vi "VoltageTest_L.vi"(0 "datain":string[](array[string])=["备注", "负载通道", "负载地址", "延时时间", "output max", "output min", "量测类型", "待测物板号"], 5 "HW CH Number":i32=4, 7 "Setup":string) -> (4 "REPORT INDECATE":string[][](array[string])=[["微安测试", "", "", "", ""], ["微安量测", "4", "0.000", "0.1", "NG"], ["微安量测", "4", "0.000", "0.1", "NG"], ["微安量测", "4", "0.000", "0.1", "NG"], ["微安量测", "4", "0.000", "0.1", "NG"]], 6 "ROW HEAD":string[](array[string]), 8 "PF":string[](array[string]), 10 "testData":string[](array[string]), 14 "数组":bool[](array[boolean]), 15 "Array":string[](array[string]))   [LabVIEW 2018]
uses:
  Subvi/Global.vi
panel:
  out "测试板数":i32=4
  # "[VoltageTest]\nExt.Name =2222222222;\nAddress =1;\nDelay Time =1;\nMAX.Spec =*;\nMin.Spec =2;\nTest Type =;\nRelayH_8Bit =0,0,0,0;\nRelayL_8Bit =0,0,0,0;\nStart board number =1;#"
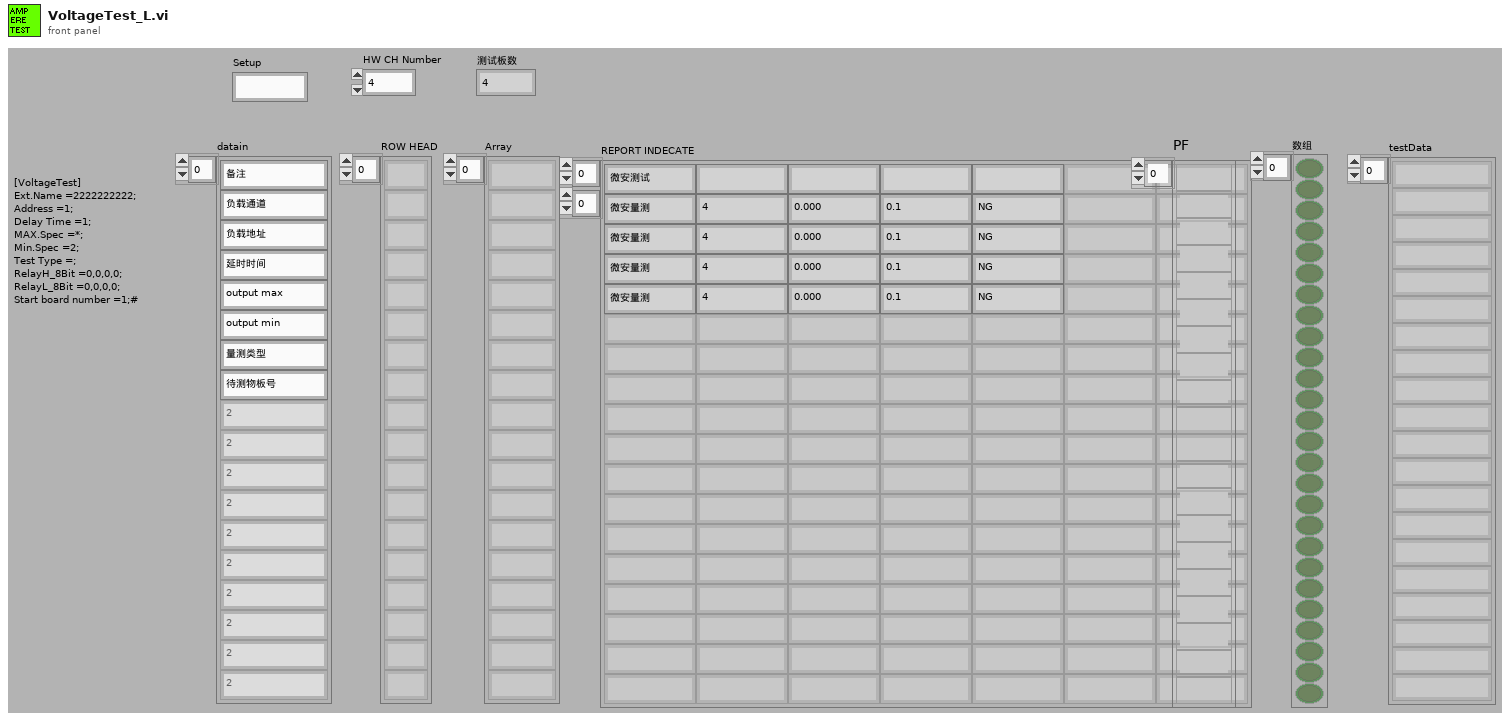
[diagram p1: front panel]
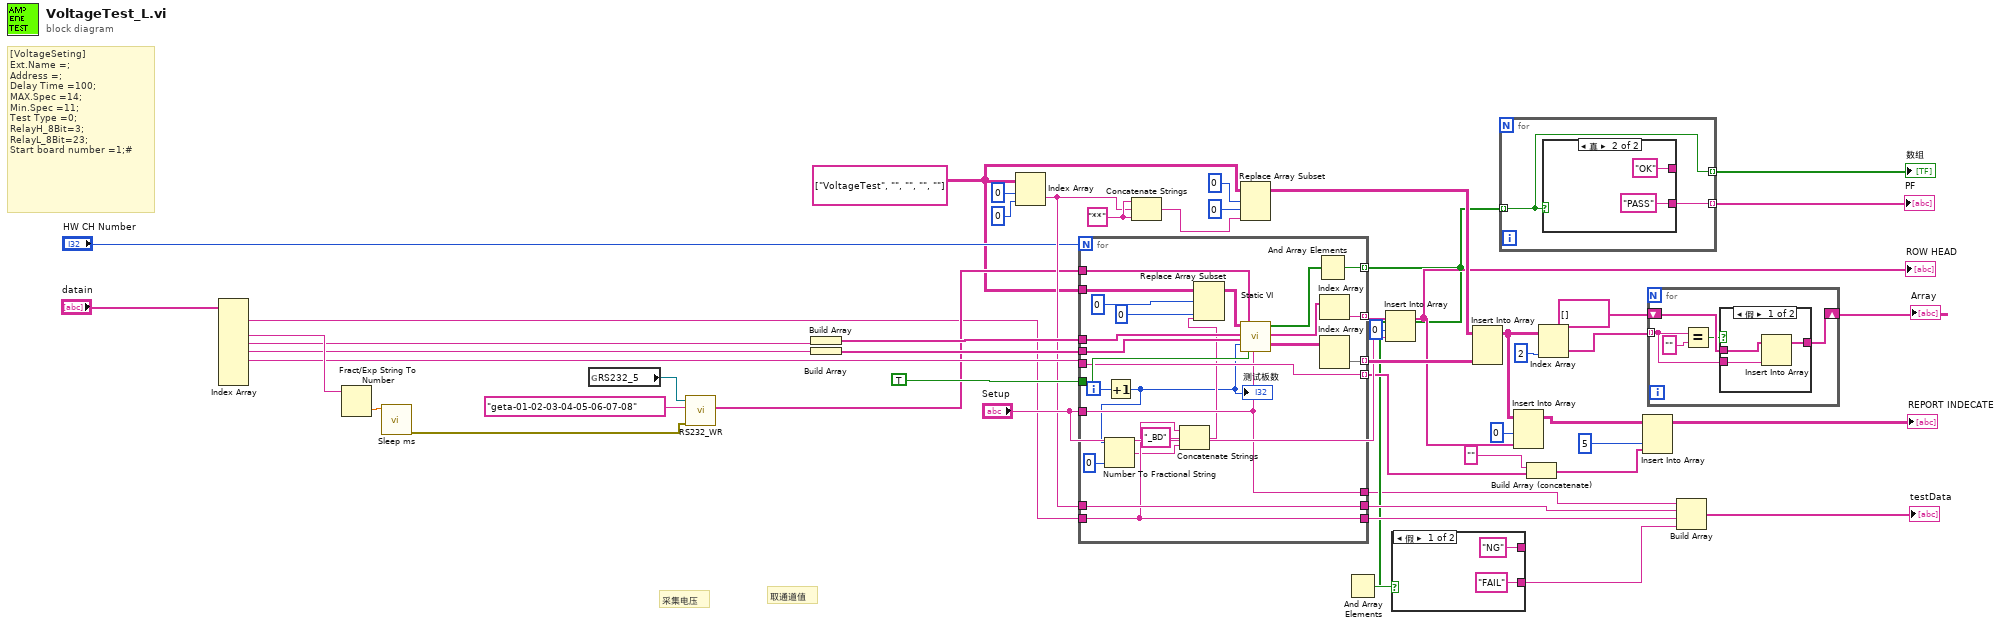
[diagram p0: block diagram]
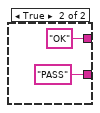
[diagram p2: hidden frame]
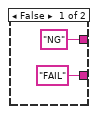
[diagram p3: hidden frame]
diagram:
  w5 = string[][] [["VoltageTest", "", "", "", ""]]
  w41 = "**" ("字符串")
  # "取通道值"
  # "采集电压"
  # "[VoltageSeting]\nExt.Name =;\nAddress =;\nDelay Time =100;\nMAX.Spec =14;\nMin.Spec =11;\nTest Type =0;\nRelayH_8Bit=3;\nRelayL_8Bit=23;\nStart board number =1;#"
  n1 = Index Array(array="datain") -> (element #1=w6:string, element #3=w44:string, element #4=w37:string, element #5=w36:string, element #6=w24:string)  [unwired: 9 in, 4 out]
  n2 = Fract/Exp String To Number(string=w44) -> (number=w2:dbl)  [unwired: 3 in, 1 out]
  n3 = call "Sleep ms.vi"("等待时间（毫秒）"=w2) -> ("error out"=w1:errorcluster)  [unwired: 10 in]
  n4 = global read "Global.vi" "RS232_5"() -> (w3:refnum<visa-resource-name>)
  n5 = call "RS232_WR.vi"("error in (no error)"=w1, "CMD"="geta-01-02-03-04-05-06-07-08", "VISA资源名称"=w3) -> ("Out data"=w7:string[])  [unwired: 6 in, 2 out]
  n6 = Build Array(w37) -> (w35:string[])
  n7 = Build Array(w36) -> (w34:string[])
  n8 = Index Array(array=w5, index (row)=0 ("索引 (行)"), index (col)=0 ("禁用的索引 (列)")) -> (element=w17:string)
  n9 = for {
    N: "HW CH Number" -> [_]
    tunnel: w7 -> [w74]
    tunnel: w35 -> [w73]
    tunnel: w34 -> [w72]
    tunnel: "Setup" -> [w62]
    tunnel: TRUE -> [w70]
    tunnel: [w69] -> w13 mode=indexing
    tunnel: [w67] -> w30 mode=indexing
    tunnel: [w65] -> w31 mode=indexing
    tunnel: w24 -> [w64]
    tunnel: [w64] -> w20 mode=indexing
    tunnel: w17 -> [w63]
    tunnel: [w63] -> w16
    tunnel: w6 -> [w54]
    tunnel: [w54] -> w15
    tunnel: [w62] -> w10
    tunnel: w5 -> [w60]
    i -> [w57]
    n10 = Increment(x=w57) -> (x+1=w51:i32)
    "测试板数" <- w51
    n11 = Number To Fractional String(number=w51, precision (6)=i16 0 ("精度(6)")) -> (F-format string=w53:string)  [unwired: 2 in]
    n12 = Concatenate Strings(w54, "_BD" ("字符串"), w53) -> (w52:string)
    n13 = Replace Array Subset(array=w60, new element=w52, index (row)=0 ("索引 (行)"), index (col)=0 ("禁用的索引 (列)")) -> (w59:string[][])
    n14 = call "Static VI.vi"("添加的数组"=w59, "Max"=w73, "Min"=w72, "板数"=w51, "INPUTSTRING"=w74, "是否为字符串对比"=w70, "SQ"=w62) -> ("P/F"=w71:bool[], "SQ out"=w68:string[], "arrauy out"=w66:string[][])  [unwired: 9 in, 1 out]
    n15 = And Array Elements(Boolean array=w71) -> (logical AND=w69:bool)
    n16 = Index Array(array=w68) -> (element=w67:string)  [unwired: 1 in]
    n17 = Index Array(array=w66) -> (element=w65:string[])  [unwired: 2 in]
  }
  n18 = Concatenate Strings(w41, w17, w41) -> (w38:string)
  n19 = Replace Array Subset(array=w5, new element=w38, index (row)=0 ("索引 (行)"), index (col)=0 ("禁用的索引 (列)")) -> (w32:string[][])
  n20 = And Array Elements(Boolean array=w13) -> (logical AND=w14:bool)
  n21 = Insert Into Array(array=w30, index=0 ("索引"), new element="Setup") -> (w26:string[])
  "ROW HEAD" <- w26
  n22 = case shown="假" w14 {
    tunnel: ["NG" "OK"] -> _
    tunnel: ["FAIL" "PASS"] -> w12
    frame False {
    }
    frame True {
    }
  }
  n23 = Insert Into Array ("数组插入")(array=w32, new element=w31) -> (w27:string[][])  [unwired: 2 in]
  n24 = for {
    tunnel: w13 -> [w79] mode=indexing
    tunnel: [w80] -> w46 mode=indexing
    tunnel: [w79] -> w9 mode=indexing
    n25 = case shown="真" w79 {
      tunnel: ["NG" "OK"] -> _
      tunnel: ["FAIL" "PASS"] -> w80
      frame False {
      }
      frame True {
      }
    }
  }
  "PF" <- w46
  "数组" <- w9
  n26 = Insert Into Array(array=w27, index (col)=0 ("禁用的索引 (列)"), new element=w26) -> (w22:string[][])  [unwired: 1 in]
  n27 = Build Array (concatenate)("" ("字符串"), w20) -> (w18:string[])
  n28 = Index Array(array=w27, index (col)=2 ("禁用的索引 (列)")) -> (element=w48:string[])  [unwired: 1 in]
  n29 = Insert Into Array(array=w22, index (col)=5 ("禁用的索引 (列)"), new element=w18) -> (→"REPORT INDECATE":string[][])  [unwired: 1 in]
  n30 = for {
    tunnel: w48 -> [w85] mode=indexing
    shift-right: [w86] -> w47
    shift-left: string[] [] ("Array") -> [w89]
    n31 = Equal?(x=w85, y="") -> (x = y?=w87:bool)
    n32 = case shown="假" w87 {
      tunnel: w89 -> [w92 w93]
      tunnel: [w91 w93] -> w86
      tunnel: w85 -> [w90 _]
      frame False {
        n33 = Insert Into Array(array=w92, new element=w90) -> (w91:string[])  [unwired: 1 in]
      }
      frame True {
      }
    }
  }
  "Array" <- w47
  n34 = Build Array(w10, w16, w15, w12) -> (→"testData":string[])
